vi "2 line get round center.vi"(1 "D":cluster{dbl, dbl}, 2 "C":cluster{dbl, dbl}, 3 "B":cluster{dbl, dbl}, 4 "A":cluster{dbl, dbl}) -> (0 "round center":cluster{dbl, dbl})   [LabVIEW 2019]
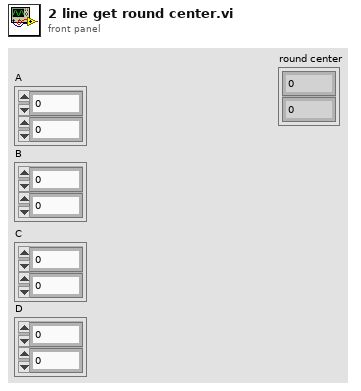
[diagram p1: front panel]
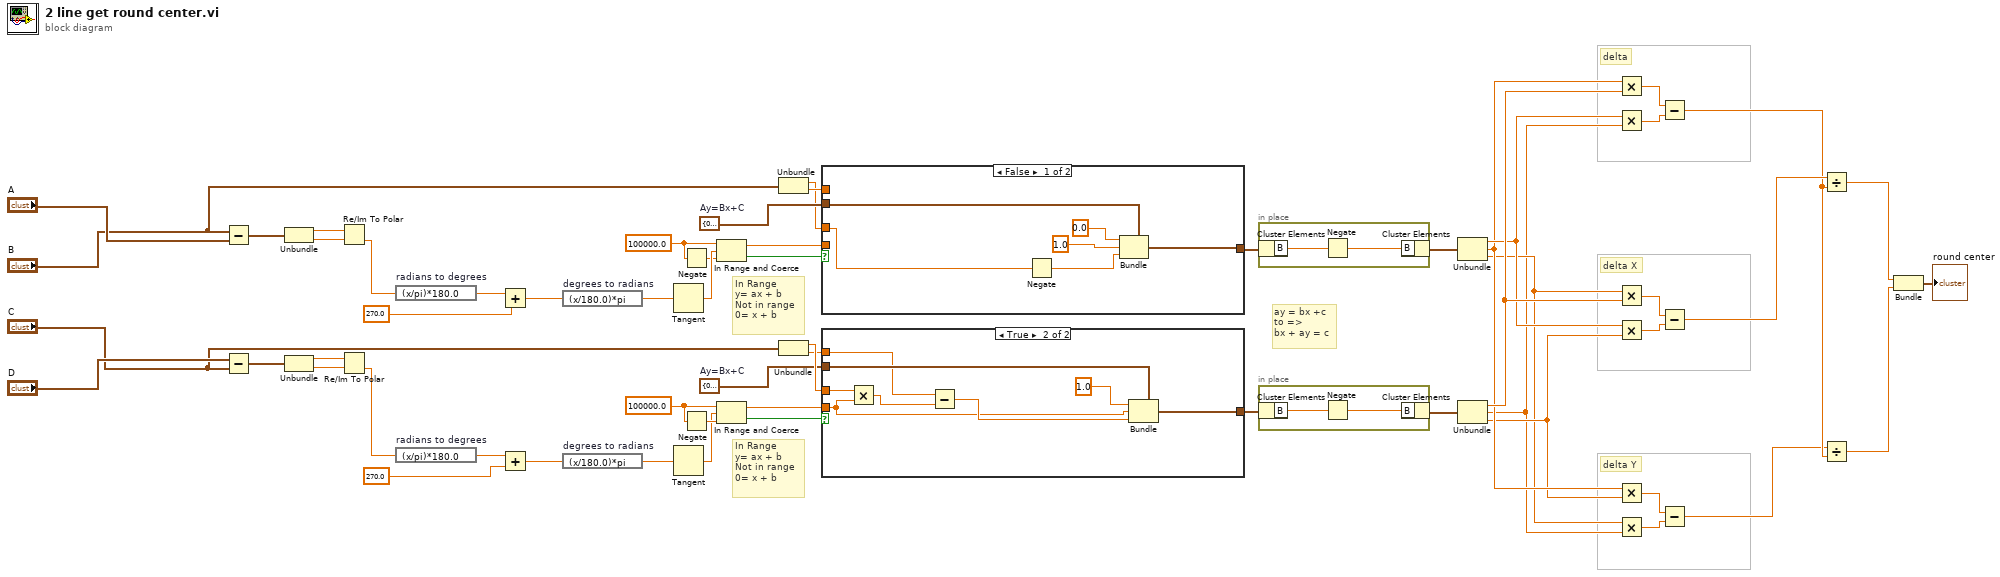
[diagram p0: block diagram]
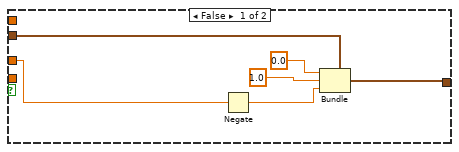
[diagram p2: hidden frame]
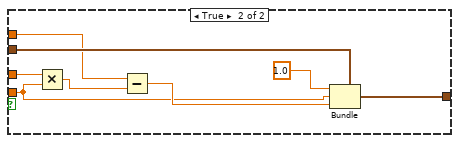
[diagram p3: hidden frame]
diagram:
  w30 = 100000.0
  w33 = cluster{"A":dbl, "B":dbl, "C":dbl} {"A"=0.0, "B"=0.0, "C"=0.0}  # Ay=Bx+C
  w46 = 100000.0
  w43 = cluster{"A":dbl, "B":dbl, "C":dbl} {"A"=0.0, "B"=0.0, "C"=0.0}  # Ay=Bx+C
  # "delta Y"
  # "delta X"
  # "delta"
  # "ay = bx +c \nto =>\nbx + ay = c"
  # "In Range \ny= ax + b\nNot in range\n0= x + b"
  # "In Range \ny= ax + b\nNot in range\n0= x + b"
  n1 = Subtract(x="B", y="A") -> (x-y=w42:cluster{dbl, dbl})
  n2 = Subtract(x="D", y="C") -> (x-y=w57:cluster{dbl, dbl})
  n3 = Unbundle(w42) -> (w56:dbl, w55:dbl)
  n4 = Unbundle(w57) -> (w54:dbl, w53:dbl)
  n5 = Re/Im To Polar(2:w55, 3:w56) -> (0:w52:dbl)  [unwired: 1 out]
  n6 = Re/Im To Polar(2:w53, 3:w54) -> (0:w23:dbl)  [unwired: 1 out]
  n7 = expression code="(x/pi)*180.0" "radians to degrees"(w52) -> (w51:dbl)
  n8 = expression code="(x/pi)*180.0" "radians to degrees"(w23) -> (w25:dbl)
  n9 = Add(x=w51, y=270.0) -> (x+y=w48:dbl)
  n10 = Add(x=w25, y=270.0) -> (x+y=w28:dbl)
  n11 = expression code="(x/180.0)*pi" "degrees to radians"(w48) -> (w49:dbl)
  n12 = expression code="(x/180.0)*pi" "degrees to radians"(w28) -> (w27:dbl)
  n13 = Tangent(1:w49) -> (0:w47:dbl)
  n14 = Tangent(1:w27) -> (0:w29:dbl)
  n15 = Negate(x=w46) -> (-x=w45:dbl)
  n16 = Negate(x=w30) -> (-x=w31:dbl)
  n17 = In Range and Coerce(upper limit=w46, x=w47, lower limit=w45) -> (coerced(x)=w39:dbl, In Range?=w44:bool)
  n18 = In Range and Coerce(upper limit=w30, x=w29, lower limit=w31) -> (coerced(x)=w35:dbl, In Range?=w32:bool)
  n19 = Unbundle("B") -> (w38:dbl, w40:dbl)
  n20 = Unbundle("C") -> (w36:dbl, w34:dbl)
  n21 = case shown="False" w44 {
    tunnel: w43 -> [w64 w72]
    tunnel: w40 -> [_ w70]
    tunnel: w39 -> [_ w66]
    tunnel: w38 -> [w60 w69]
    tunnel: [w59 w65] -> w22
    frame False {
      n22 = Negate(x=w60) -> (-x=w61:dbl)
      n23 = Bundle(cluster=w64, "A"=0.0, "B"=1.0, "C"=w61) -> (w59:cluster{"A":dbl, "B":dbl, "C":dbl})
    }
    frame True {
      n24 = Multiply(x=w69, y=w66) -> (x*y=w68:dbl)
      n25 = Subtract(x=w70, y=w68) -> (x-y=w67:dbl)
      n26 = Bundle(cluster=w72, "A"=1.0, "B"=w66, "C"=w67) -> (w65:cluster{"A":dbl, "B":dbl, "C":dbl})
    }
  }
  n27 = case shown="True" w32 {
    tunnel: w33 -> [w78 w86]
    tunnel: w34 -> [_ w84]
    tunnel: w35 -> [_ w80]
    tunnel: w36 -> [w74 w83]
    tunnel: [w73 w79] -> w21
    frame False {
      n28 = Negate(x=w74) -> (-x=w75:dbl)
      n29 = Bundle(cluster=w78, "A"=0.0, "B"=1.0, "C"=w75) -> (w73:cluster{"A":dbl, "B":dbl, "C":dbl})
    }
    frame True {
      n30 = Multiply(x=w83, y=w80) -> (x*y=w82:dbl)
      n31 = Subtract(x=w84, y=w82) -> (x-y=w81:dbl)
      n32 = Bundle(cluster=w86, "A"=1.0, "B"=w80, "C"=w81) -> (w79:cluster{"A":dbl, "B":dbl, "C":dbl})
    }
  }
  n33 = in-place {
    n34 = in-place-cluster #1(w22) -> ("B"=w88:dbl)
    n35 = Negate(x=w88) -> (-x=w87:dbl)
    n36 = in-place-cluster #1("B"=w87) -> (w20:cluster{"A":dbl, "B":dbl, "C":dbl})
  }
  n37 = in-place {
    n38 = in-place-cluster #2(w21) -> ("B"=w90:dbl)
    n39 = Negate(x=w90) -> (-x=w89:dbl)
    n40 = in-place-cluster #2("B"=w89) -> (w19:cluster{"A":dbl, "B":dbl, "C":dbl})
  }
  n41 = Unbundle(w20) -> ("A"=w11:dbl, "B"=w10:dbl, "C"=w8:dbl)
  n42 = Unbundle(w19) -> ("A"=w14:dbl, "B"=w7:dbl, "C"=w9:dbl)
  n43 = Multiply(x=w10, y=w14) -> (x*y=w18:dbl)
  n44 = Multiply(x=w11, y=w7) -> (x*y=w17:dbl)
  n45 = Multiply(x=w8, y=w14) -> (x*y=w15:dbl)
  n46 = Multiply(x=w11, y=w9) -> (x*y=w16:dbl)
  n47 = Multiply(x=w10, y=w9) -> (x*y=w13:dbl)
  n48 = Multiply(x=w8, y=w7) -> (x*y=w12:dbl)
  n49 = Subtract(x=w18, y=w17) -> (x-y=w5:dbl)
  n50 = Subtract(x=w15, y=w16) -> (x-y=w6:dbl)
  n51 = Subtract(x=w13, y=w12) -> (x-y=w4:dbl)
  n52 = Divide(x=w6, y=w5) -> (x/y=w3:dbl)
  n53 = Divide(x=w4, y=w5) -> (x/y=w2:dbl)
  n54 = Bundle(w3, w2) -> (→"round center":cluster{dbl, dbl})  [unwired: 1 in]
